vi "SW_Write_Cage's_Geometrical_Parameter.vi"(8 "Error In":errorcluster, 9 "Parameter value":variant, 10 "Parameter to update":enum16{"None", "Cage diameter/size"}(ring), 11 "Geometry in":T1 {"Cage type" items=["Round", "Square", "Donut-maze", "T-maze", "Sociability maze", ""]}) -> (0 "Error Out":errorcluster, 3 "Geometry out":T1 {"Cage type" items=["Round", "Square", "Donut-maze", "T-maze", "Sociability maze", ""]})   [LabVIEW 2018, in "Common_Resources.lvlib"]
uses:
  Common/Typedefs/CTL_Segmented_plot_parameters_2.ctl
  Libraries/Cage Diagram/Typedefs/CTL_Cage_type.ctl
  Controls/CTL_Cage_all_segmentation_params_set.ctl
  Common/Typedefs/CTL_Segmented_plot_parameters_2_(round_d1).ctl
  Common_Resources.lvlib
  Libraries/Cage Diagram/Cage Diagram.lvlib
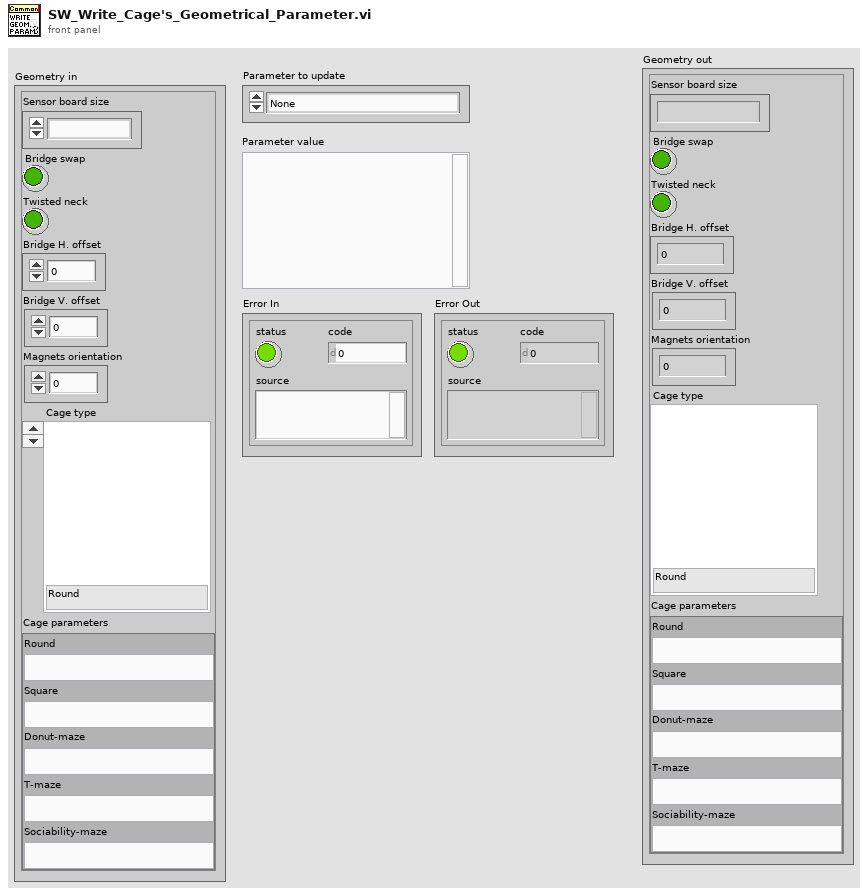
[diagram p1: front panel]
types:
  T1 = typedef "Common_Resources.lvlib/CTL_Segmented_plot_parameters_2.ctl" = cluster{"Sensor board size":enum16{"", "Large"}, "Bridge swap":bool, "Twisted neck":bool, "Bridge H. offset":sgl, "Bridge V. offset":sgl, "Magnets orientation":sgl, "Cage type":T2, "Cage parameters":T3}
  T2 = typedef "Cage Diagram.lvlib/CTL_Cage_type.ctl" = u16
  T3 = typedef "Common_Resources.lvlib/CTL_Cage_all_segmentation_params_set.ctl" = cluster{"Round":variant, "Square":variant, "Donut-maze":variant, "T-maze":variant, "Sociability-maze":variant}
  T4 = typedef "Common_Resources.lvlib/CTL_Segmented_plot_parameters_2_(round_d1).ctl" = cluster{"Cage diameter, mm":u16, "Starting angle BORDER":i16, "Starting angle MIDFIELD":i16, "Radius, mm MIDFIELD":u16, "Radius, mm CENTER":u16, "N segments BORDER":u8, "N segments MIDFIELD":u8, "R-gap, mm":sgl}
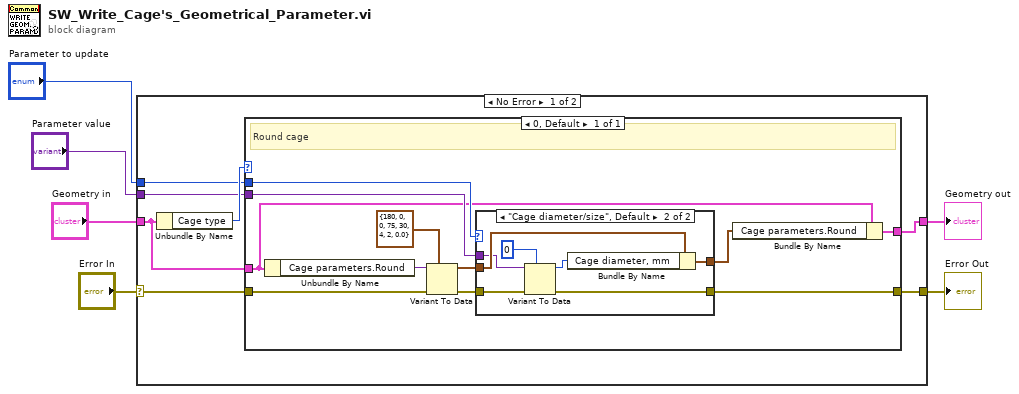
[diagram p0: block diagram]
diagram:
  n1 = case shown="No Error" "Error In" {
    selector: "Error In" -> [w10 w34]
    tunnel: "Geometry in" -> [w12 w35]
    tunnel: "Parameter value" -> [w9 _]
    tunnel: "Parameter to update" -> [w11 _]
    tunnel: [w8 w34] -> w2
    tunnel: [w7 w35] -> w1
    frame No Error {
      n2 = Unbundle By Name(w12) -> ("Cage type"=w13:T2)
      n3 = case shown="0, Default" w13 {
        tunnel: w12 -> [w16]
        tunnel: w11 -> [w21]
        tunnel: w10 -> [w22]
        tunnel: w9 -> [w18]
        tunnel: [w17] -> w8
        tunnel: [w14] -> w7
        frame 0, Default {
          # "Round cage"
          n4 = Unbundle By Name(w16) -> ("Cage parameters.Round"=w24:variant)
          n5 = Variant To Data(error in=w22, type=T4 {"Cage diameter, mm"=180, "Starting angle BORDER"=0, "Starting angle MIDFIELD"=0, "Radius, mm MIDFIELD"=75, "Radius, mm CENTER"=30, "N segments BORDER"=4, "N segments MIDFIELD"=2, "R-gap, mm"=0.0} ("Radial segmentation parameters"), Variant=w24) -> (data=w19:T4, error out=w20:errorcluster)
          n6 = case shown="\"Cage diameter/size\", Default" w21 {
            tunnel: w20 -> [w25 w31]
            tunnel: w19 -> [w26 w33]
            tunnel: w18 -> [_ w29]
            tunnel: [w25 w28] -> w17
            tunnel: [w26 w27] -> w15
            frame "None" {
            }
            frame "Cage diameter/size", Default {
              n7 = Variant To Data(error in=w31, type=u16 0 ("Cage diameter, mm"), Variant=w29) -> (data=w30:u16, error out=w28:errorcluster)
              n8 = Bundle By Name(cluster=w33, "Cage diameter, mm"=w30) -> (w27:T4)
            }
          }
          n9 = Bundle By Name(cluster=w16, "Cage parameters.Round"=w15) -> (w14:T1)
        }
      }
    }
    frame Error {
    }
  }
  "Error Out" <- w2
  "Geometry out" <- w1
